vi "Run.vi"(8 "error in":errorcluster caption="entrée d'erreur", 11 "lfw_people.lvclass":refnum<class "lfw_people.lvclass">) -> (0 "error out":errorcluster caption="sortie d'erreur", 2 "Data":T1, 3 "lfw_people.lvclass":refnum<class "lfw_people.lvclass">)   [LabVIEW 2020, in "lfw_people.lvclass"]
doc: "Returns : \n\n- data : numpy array of shape (13233, 62, 47)\nEach row is a face image corresponding to one of the 5749 people in the dataset. Changing the slice_ or resize parameters will change the shape of the output.\n\n- target : numpy array of shape (13233,)\nLabels associated to each face image. Those labels range from 0-5748 and correspond to the person IDs."
uses:
  lfw_people.lvclass
  lfw_people.lvclass/lfw_people.ctl
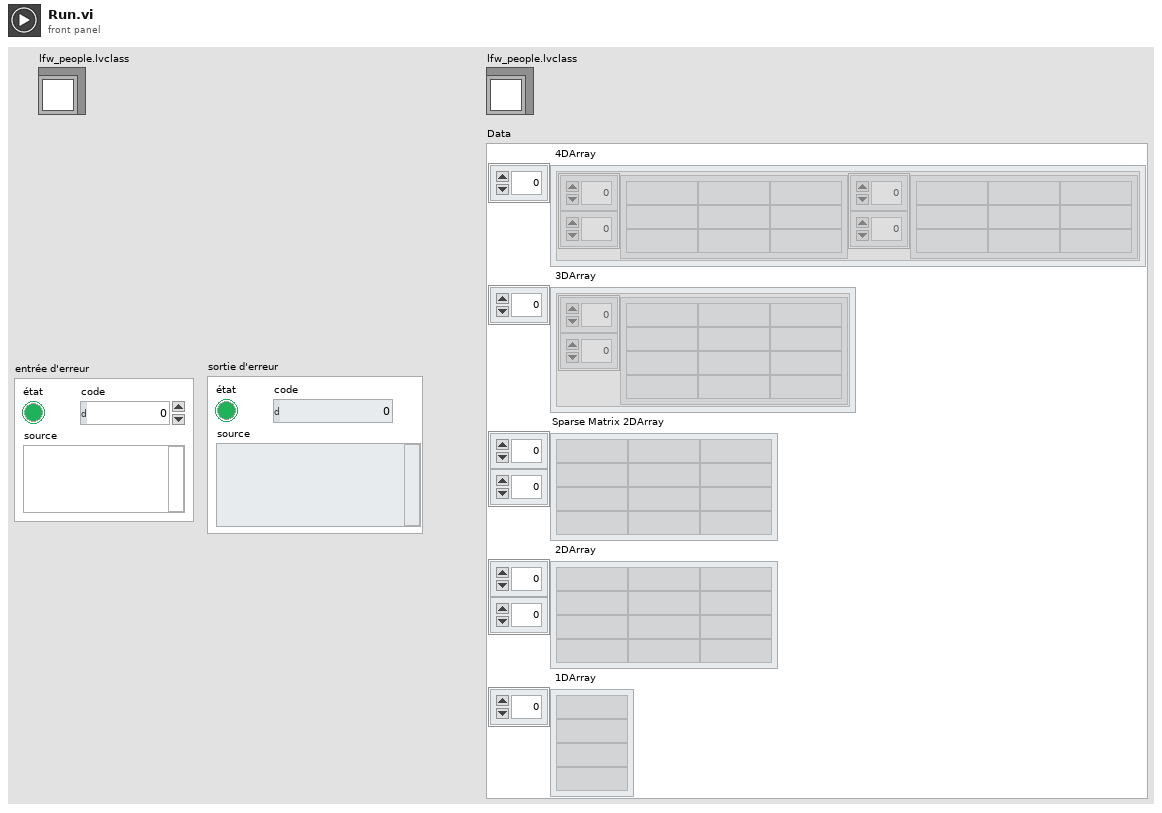
[diagram p1: front panel]
types:
  T1 = cluster{" 4DArray":cluster{"1":string[][], "2":string[][]}[], " 3DArray":cluster{"Tableau":string[][]}[], "Sparse Matrix 2DArray":string[][], " 2DArray":string[][], " 1DArray":string[]}
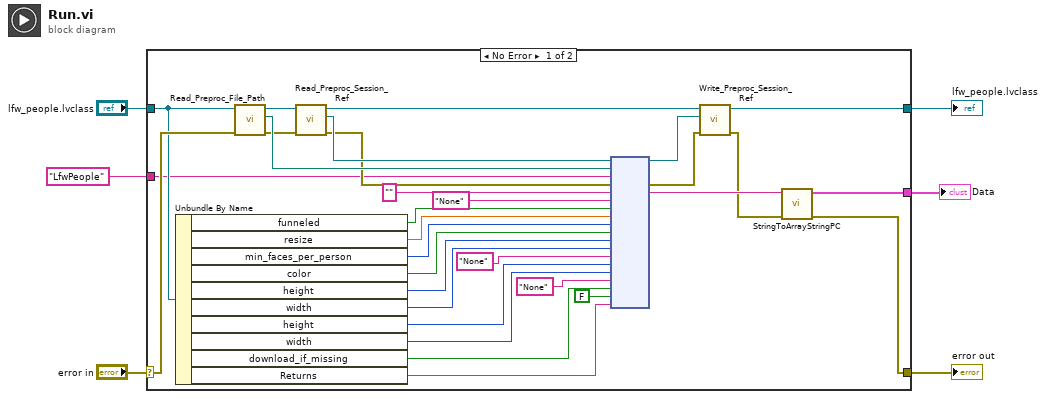
[diagram p0: block diagram]
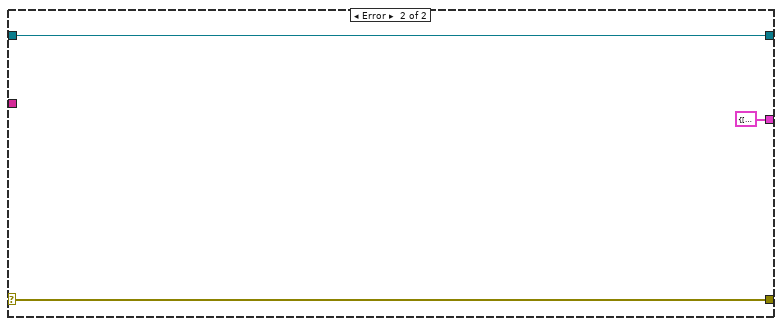
[diagram p2: hidden frame]
diagram:
  n1 = case shown="No Error" "error in" {
    selector: "error in" -> [w30 w40]
    tunnel: [w8 w40] -> w5
    tunnel: [w11 w39] -> w3
    tunnel: "lfw_people.lvclass" -> [w29 w39]
    tunnel: "LfwPeople" -> [w28 _]
    tunnel: [w7 T1 {" 4DArray"=[], " 3DArray"=[], "Sparse Matrix 2DArray"=[], " 2DArray"=[], " 1DArray"=[]} ("Data")] -> w1
    frame No Error {
      n2 = Unbundle By Name(w29) -> ("funneled"=w27:bool, "resize"=w26:dbl, "min_faces_per_person"=w24:i32, "color"=w23:bool, "height"=w22:u32, "width"=w21:u32, "height"=w19:u32, "width"=w18:u32, "download_if_missing"=w16:bool, "Returns"=w12:string)
      n3 = call-dynamic "Read_Preproc_File_Path.vi"("error in (no error)"=w30, "Python in"=w29) -> ("error out"=w32:errorcluster, "File_Path"=w35:path, "Python out"=w37:refnum<class "lfw_people.lvclass">)  [unwired: 7 in]
      n4 = call-dynamic "Read_Preproc_Session_Ref.vi"("error in (no error)"=w32, "Python in"=w37) -> ("error out"=w33:errorcluster, "Session_ref"=w34:refnum<k35>, "Python out"=w36:refnum<class "lfw_people.lvclass">)  [unwired: 7 in]
      n5 = node(w34, w35, w28, w33, "", "None", w27, w26, w24, w23, w22, w21, "None", w19, w18, "None", w16, FALSE, w12) -> (w14:refnum<k35>, w13:errorcluster, w10:string)  [unwired: 14 in, 2 out]
      n6 = call-dynamic "Write_Preproc_Session_Ref.vi"("error in (no error)"=w13, "Session_ref"=w14, "Python in"=w36) -> ("error out"=w9:errorcluster, "Python out"=w11:refnum<class "lfw_people.lvclass">)  [unwired: 7 in]
      n7 = call "StringToArrayStringPC.vi"("sortie d'erreur"=w9, "Return value"=w10) -> ("sortie d'erreur"=w8:errorcluster, "Data"=w7:T1)  [unwired: 8 in]
    }
    frame Error {
    }
  }
  "error out" <- w5
  "lfw_people.lvclass" <- w3
  "Data" <- w1
